vi "Place Hatch Level 1.vi"   [LabVIEW 2018]
uses:
  SubSystems/Hatch Panel Intake/Hatch Panel Intake Global.vi
  SubSystems/Lift/Lift Global.vi
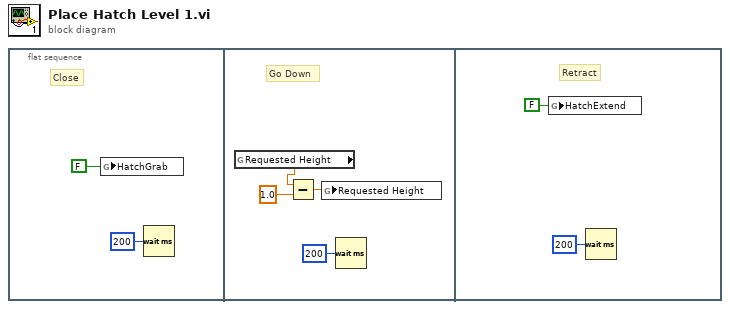
[diagram p0: block diagram]
diagram:
  n1 = flat-sequence {
    frame #0 {
      # "Close"
      n2 = global write "Hatch Panel Intake Global.vi" "HatchGrab"(FALSE ("HatchExtend")) -> ()
      n3 = Wait (ms)(milliseconds to wait=u32 200) -> ()  [unwired: 1 out]
    }
    frame #1 {
      # "Go Down"
      n4 = global read "Lift Global.vi" "Requested Height"() -> (w5:dbl)
      n5 = Subtract(x=w5, y=1.0) -> (x-y=w6:dbl)
      n6 = global write "Lift Global.vi" "Requested Height"(w6) -> ()
      n7 = Wait (ms)(milliseconds to wait=u32 200) -> ()  [unwired: 1 out]
    }
    frame #2 {
      # "Retract"
      n8 = global write "Hatch Panel Intake Global.vi" "HatchExtend"(FALSE ("HatchExtend")) -> ()
      n9 = Wait (ms)(milliseconds to wait=u32 200) -> ()  [unwired: 1 out]
    }
  }
